vi "Print.vi"(8 "error in (no error)":errorcluster, 11 "Message Response in":refnum<class "Message Response.lvclass">) -> (0 "error out":errorcluster, 2 "String":string, 3 "Message Response out":refnum<class "Message Response.lvclass">)   [LabVIEW 2016, in "WebSocket Networking.lvlib" / "Message Response.lvclass"]
doc: "--\nCopyright © 2017 Composed SystemsI All rights reserved.\n\nAuthor: Jon McBee <jon.mcbee@composed.io>\n\nThis library is provided \"AS IS\" ,WITHOUT WARRANTIES OR\nCONDITIONS OF ANY KIND, either express or implied.\n\nComposed Systems -- composed.io\n\nStream 0.0.1.1\nJon McBee - Composed Systems\nCopyright (c) 2017, Composed Systems"
uses:
  <userlib>/Common Components/WebSocket Networking/Message Response/Message Response.lvclass
  <userlib>/Composed Systems/Stream/Mediator/Classes/Message Data Interface/Data Message Interface.lvclass
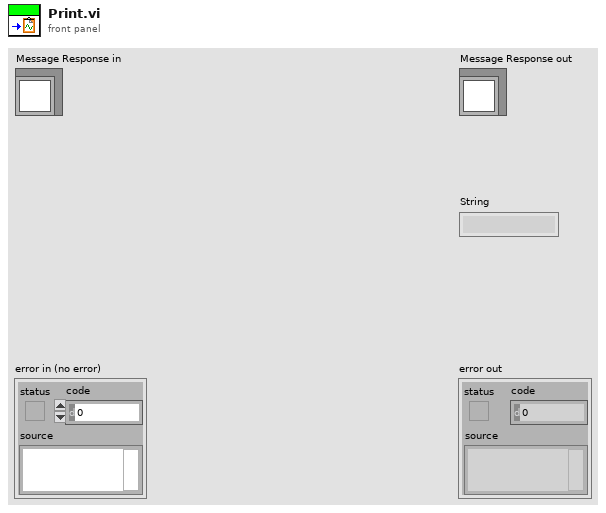
[diagram p1: front panel]
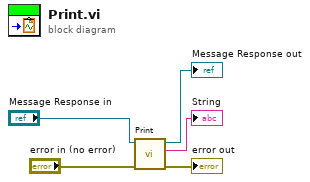
[diagram p0: block diagram]
diagram:
  n1 = call-parent "Print.vi"("error in (no error)"="error in (no error)", "Message Interface in"="Message Response in") -> ("error out"=→"error out":errorcluster, "String"=→"String":string, "Message Interface out"=→"Message Response out":refnum<class "Message Response.lvclass">)  [unwired: 7 in]
